vi "Fire User Event - Stop.vi"(8 "error in (no error)":errorcluster, 11 "User events":T1) -> (0 "error out":errorcluster)   [LabVIEW 2020, in "User Event - Stop.lvlib"]
doc: "Send the Stop event to stop the Event Handling Loop."
uses:
  User Event - Stop.lvlib
  controls/Wake HL data -- cluster.ctl
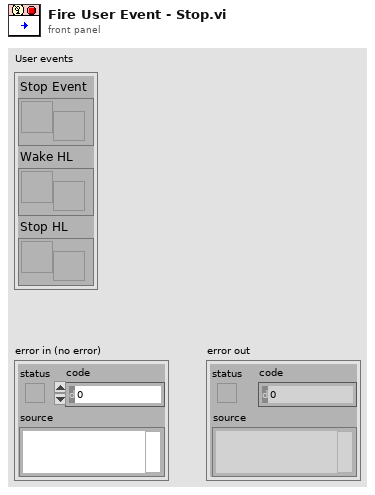
[diagram p1: front panel]
types:
  T1 = cluster{"Stop Event":refnum<user-event>, "Wake HL":refnum<user-event>, "Stop HL":refnum<user-event>}
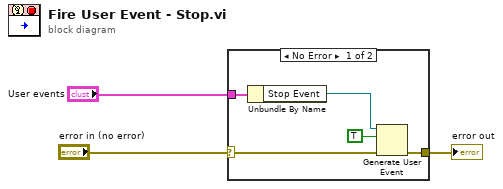
[diagram p0: block diagram]
diagram:
  n1 = case shown="No Error" "error in (no error)" {
    selector: "error in (no error)" -> [w6 w9]
    tunnel: [w7 w9] -> w3
    tunnel: "User events" -> [w5 _]
    frame No Error {
      n2 = Unbundle By Name(w5) -> ("Stop Event"=w4:refnum<user-event>)
      n3 = Generate User Event(user event=w4, event data cluster=TRUE ("event data"), error in=w6) -> (error out=w7:errorcluster)  [unwired: 1 in, 1 out]
    }
    frame Error {
    }
  }
  "error out" <- w3
